vi "create aggregate stats.vi"(4 "US data":T1, 6 "Aggregate name":string, 7 "country indexes of aggregate":i32[](array[numeric]), 8 "populations US":i32[](array[numeric]), 9 "Populations global":i32[](array[numeric]), 10 "global deaths":string[][](array[string]), 11 "global cases":string[][](array[string])) -> (1 "population":i64, 2 "deaths array array":string[](array[string]), 3 "cases array":string[](array[string]))   [LabVIEW 2019]
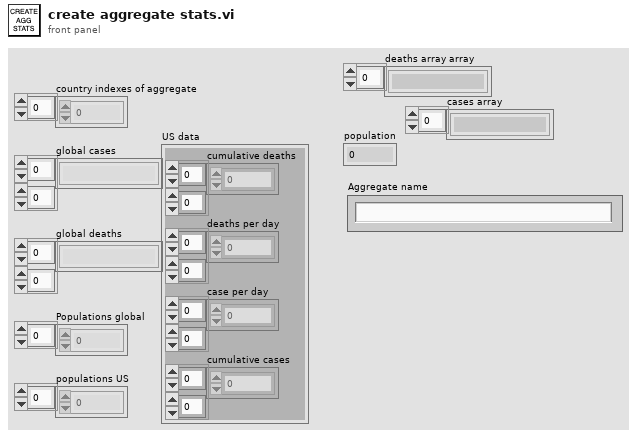
[diagram p1: front panel]
types:
  T1 = cluster{"cumulative deaths":i32[][], "deaths per day":i32[][], "case per day":i32[][], "cumulative cases":i32[][]}
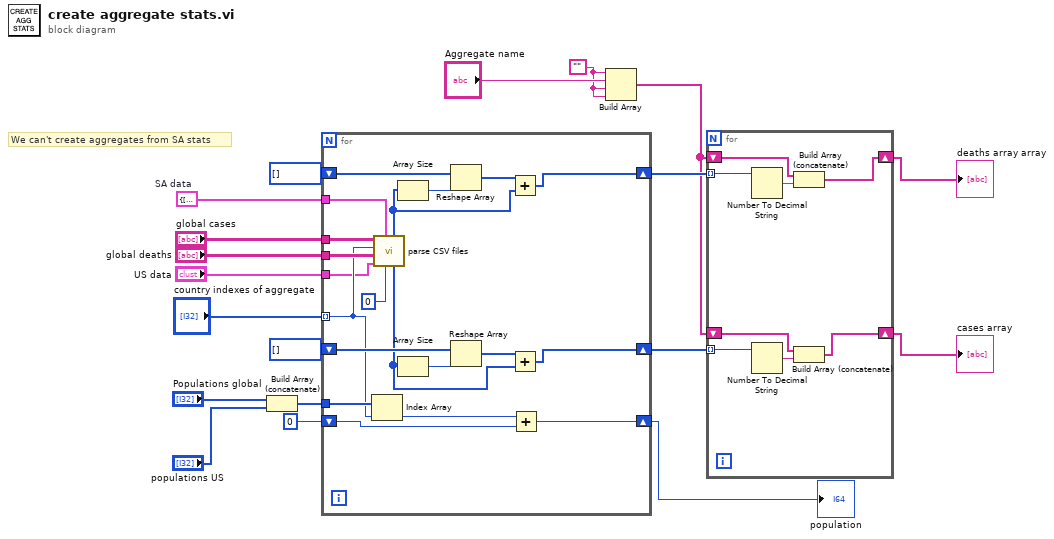
[diagram p0: block diagram]
diagram:
  w1 = T1 {"cumulative deaths"=[], "deaths per day"=[], "case per day"=[], "cumulative cases"=[]}  # SA data
  w7 = ""
  # "We can't create aggregates from SA stats"
  n1 = Build Array (concatenate)("Populations global", "populations US") -> (w3:i32[])
  n2 = for {
    tunnel: "global deaths" -> [w39]
    tunnel: "global cases" -> [w38]
    tunnel: "country indexes of aggregate" -> [w25] mode=indexing
    shift-right: [w32] -> w12
    shift-left: i32[] [] -> [w34]
    shift-right: [w31] -> w11
    shift-left: i32[] [] -> [w29]
    tunnel: w3 -> [w26]
    shift-right: [w23] -> w10
    shift-left: i64 0 -> [w22]
    tunnel: "US data" -> [w21]
    tunnel: w1 -> [w20]
    n3 = Index Array(array=w26, index=w25) -> (element=w24:i32)
    n4 = call "parse CSV files.vi"("threshold cases"=u32 0, "SA data"=w20, "US data"=w21, "deaths CSV"=w39, "country index"=w25, "cases CSV"=w38) -> ("cumulative cases"=w27:i32[], "cumulative deaths"=w35:i32[])  [unwired: 4 out]
    n5 = Array Size(array=w35) -> (size(s)=w36:i32)
    n6 = Array Size(array=w27) -> (size(s)=w28:i32)
    n7 = Reshape Array(w34, w36) -> (w33:i32[])
    n8 = Reshape Array(w29, w28) -> (w30:i32[])
    n9 = Add(x=w33, y=w35) -> (x+y=w32:i32[])
    n10 = Add(x=w30, y=w27) -> (x+y=w31:i32[])
    n11 = Add(x=w24, y=w22) -> (x+y=w23:i64)
  }
  "population" <- w10
  n12 = Build Array(w7, "Aggregate name", w7, w7) -> (w8:string[])
  n13 = for {
    tunnel: w12 -> [w47] mode=indexing
    shift-right: [w43] -> w5
    shift-left: w8 -> [w44]
    tunnel: w11 -> [w46] mode=indexing
    shift-right: [w40] -> w6
    shift-left: w8 -> [w42]
    n14 = Number To Decimal String(number=w47) -> (decimal integer string=w45:string)  [unwired: 1 in]
    n15 = Number To Decimal String(number=w46) -> (decimal integer string=w41:string)  [unwired: 1 in]
    n16 = Build Array (concatenate)(w44, w45) -> (w43:string[])
    n17 = Build Array (concatenate)(w42, w41) -> (w40:string[])
  }
  "deaths array array" <- w5
  "cases array" <- w6
